vi "Check for Removed Plugin and Prune Subpanel.vi"(8 "error in (no error)":errorcluster, 11 "CIF_UI in":refnum<class "CIF_UI.lvclass">) -> (0 "error out":errorcluster, 3 "CIF_UI out":refnum<class "CIF_UI.lvclass">)   [LabVIEW 2021, in "CIF_UI.lvclass"]
uses:
  CIF_UI.lvclass
  CIF_UI.lvclass/CIF_UI.ctl
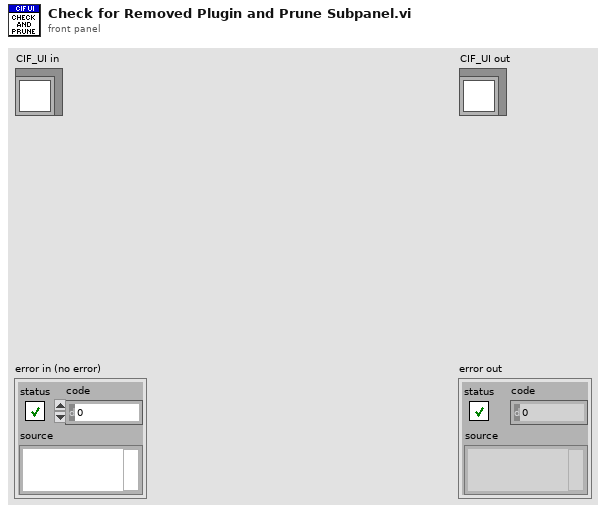
[diagram p1: front panel]
types:
  T1 = typedef "CIF_UI.lvclass/Plugin Connection Map.ctl" = map{string, T2}
  T2 = typedef "CIF_UI.lvclass/Plugin Connections.ctl" = cluster{"gRPC ID":T3, "Plugin Info":T4}
  T3 = typedef "grpc-lvsupport-release.lvlib/grpcId.ctl" = u64
  T4 = typedef "CIF_UI.lvclass/PluginInfo.ctl" = cluster{"Name":string, "Type":string, "grpc_port":i32, "Version":T5, "Node Status":T6}
  T5 = typedef "CIF_UI.lvclass/Version.ctl" = cluster{"Major":i32, "Minor":i32, "Fix":i32}
  T6 = typedef "CIFCoreCommon.lvlib/gRPC Reported Plugin Status.ctl" = cluster{"State":T7, "Timing Statistics (us)":T8, "FIFO Statistics (us)":T10, "error":T11, "Monitor Doubles":T12, "Monitor U64":T13, "Monitor I64":T14}
  T7 = typedef "CIFCoreCommon.lvlib/Plugin State.ctl" = enum32{"Null", "Creating", "Listening", "Running", "CleaningUp", "Destroying"}
  T8 = typedef "CIFCoreCommon.lvlib/Timing Statistics.ctl" = cluster{"Period":T9, "Wake Error":T9, "Execute":T9, "Housekeep":T9, "Idle":T9, "Cleanup":T9, "Custom 1 (custom units)":T9, "Custom 2 (custom units)":T9}
  T9 = typedef "CIFCoreCommon.lvlib/Timing Stats Base.ctl" = cluster{"Max":i64, "Avg":dbl, "Min":i64}
  T10 = typedef "CIFCoreCommon.lvlib/FIFO Statistics.ctl" = cluster{"From T0":T9, "From Previous Plugin":T9, "Output Error":T9}
  T11 = typedef "CIFCoreCommon.lvlib/Simple Error.ctl" = cluster{"status":bool, "code":i32}
  T12 = typedef "CIFCoreCommon.lvlib/Monitor Doubles.ctl" = cluster{"1":dbl, "2":dbl, "3":dbl, "4":dbl}
  T13 = typedef "CIFCoreCommon.lvlib/Monitor U64.ctl" = cluster{"1":u64, "2":u64, "3":u64, "4":u64}
  T14 = typedef "CIFCoreCommon.lvlib/Monitor I64.ctl" = cluster{"1":i64, "2":i64, "3":i64, "4":i64}
  T15 = typedef "CIF_UI.lvclass/Plugin Subpanel Map.ctl" = map{i32, T16}
  T16 = typedef "CIF_UI.lvclass/Subpanel Data.ctl" = cluster{"VI Reference":refnum<vi>, "Plugin Subpanel Events":T17}
  T17 = typedef "CIF_UI.lvclass/Plugin Subpanel Events.ctl" = cluster{"Plugin Shutdown":refnum<user-event>}
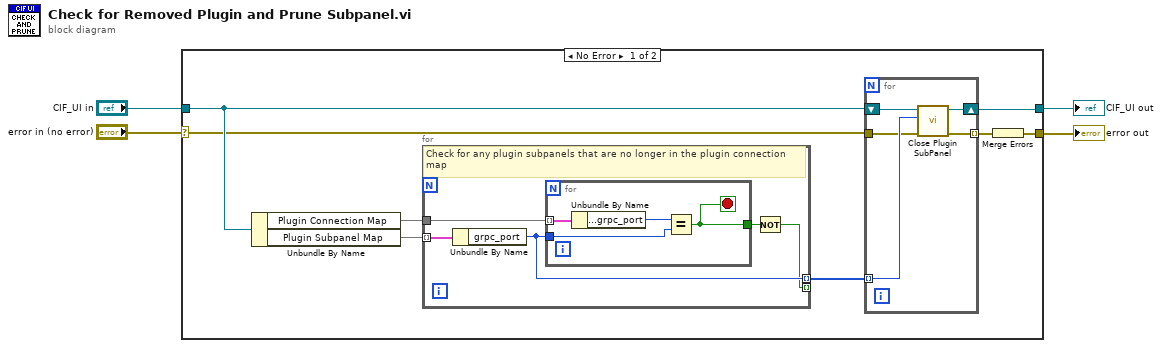
[diagram p0: block diagram]
diagram:
  n1 = case shown="No Error" "error in (no error)" {
    selector: "error in (no error)" -> [w10 w28]
    tunnel: [w5 w28] -> w3
    tunnel: [w9 w27] -> w1
    tunnel: "CIF_UI in" -> [w11 w27]
    frame No Error {
      n2 = Unbundle By Name(w11) -> ("Plugin Connection Map"=w8:T1, "Plugin Subpanel Map"=w12:T15)
      n3 = for {
        tunnel: w12 -> [w22] mode=indexing
        tunnel: w8 -> [w21]
        tunnel: [w20] -> w7 mode=indexing if=w18
        tunnel: [w18] -> _ mode=indexing
        # "Check for any plugin subpanels that are no longer in the plugin connection map"
        n4 = Unbundle By Name(w22) -> ("grpc_port"=w20:i32)
        n5 = for {
          tunnel: w20 -> [w24]
          tunnel: w21 -> [w26] mode=indexing
          tunnel: [w23] -> w19
          stop <- w23 stop-if-true
          n6 = Unbundle By Name(w26) -> ("Plugin Connections.Plugin Info.grpc_port"=w25:i32)
          n7 = Equal?(x=w25, y=w24) -> (x = y?=w23:bool)
        }
        n8 = Not(x=w19) -> (.not. x?=w18:bool)
      }
      n9 = for {
        shift-right: [w16] -> w9
        shift-left: w11 -> [w17]
        tunnel: w7 -> [w15] mode=indexing
        tunnel: w10 -> [w14]
        tunnel: [w13] -> w6 mode=indexing
        n10 = call "Close Plugin SubPanel.vi"("error in (no error)"=w14, "gRPC Port"=w15, "CIF_UI in"=w17) -> ("error out"=w13:errorcluster, "CIF_UI out"=w16:refnum<class "CIF_UI.lvclass">)  [unwired: 7 in]
      }
      n11 = Merge Errors(w6) -> (w5:errorcluster)
    }
    frame Error {
    }
  }
  "error out" <- w3
  "CIF_UI out" <- w1
